vi "Write TAG (SubVI).vi"(11 "element":T1) -> (0 "error out":errorcluster)   [LabVIEW 2017]
uses:
  Vibration.ctl
  <vilib>/Skyline/Tag/Shared/typedefs/DataType.ctl
  <vilib>/Skyline/Tag/Wrapper/Wrapper AMQP_class/Open Tag AMQP.vi
  <vilib>/Skyline/Tag/Wrapper/Wrapper_class/Generate Tag Cluster (DBL) 2.vi
  <vilib>/Skyline/Tag/Wrapper/Wrapper_class/Generate Tag Cluster (Boolean) 2.vi
  <vilib>/Skyline/Tag/Wrapper/Wrapper_class/Close Tag (Multiple).vi
  <vilib>/Skyline/Tag/Shared/NI Skyline Tag.lvlib
  <vilib>/Skyline/Tag/Wrapper/Wrapper_class/NI Skyline Tag.lvclass
  <vilib>/Skyline/Tag/Wrapper/Wrapper AMQP_class/NI Skyline Tag AMQP.lvclass
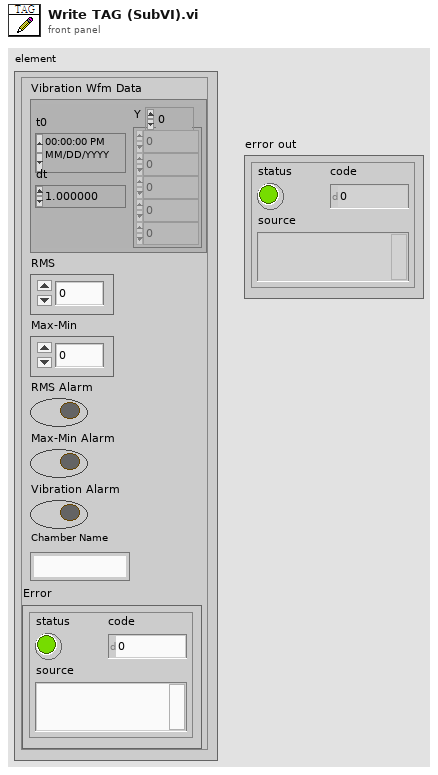
[diagram p1: front panel]
types:
  T1 = typedef "Vibration.ctl" = cluster{"Vibration Wfm Data":waveform(dbl), "RMS":dbl, "Max-Min":dbl, "RMS Alarm":bool, "Max-Min Alarm":bool, "Vibration Alarm":bool, "Chamber Name":string, "Error":errorcluster}
  T2 = typedef "NI Skyline Tag.lvlib/DataType.ctl" = enum32{"Double", "I32", "String", "Boolean", "U64", "Timestamp"}
  T3 = typedef "NI Skyline Tag.lvclass/Tag Value Cluster Wrapper.ctl" = cluster{"Configuration":refnum<class "NI Skyline Configuration.lvclass">, "Tag Cluster":T4}
  T4 = typedef "NI Skyline Tag.lvlib/Tag Value Cluster.ctl" = cluster{"Path":string, "Data Type":T2, "Value":string, "Time Stamp":timestamp}
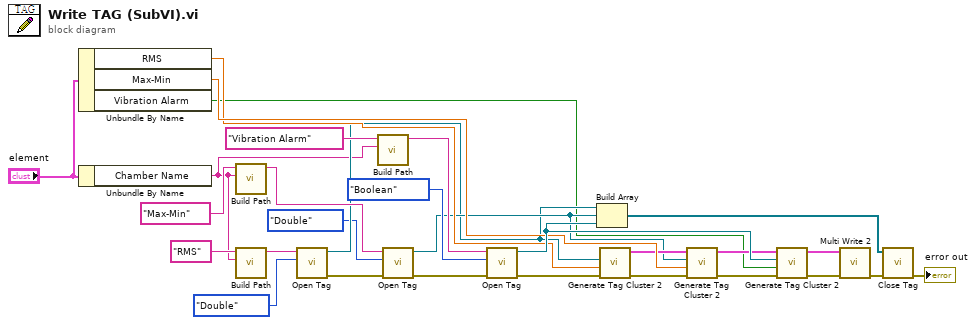
[diagram p0: block diagram]
diagram:
  n1 = Unbundle By Name("element") -> ("RMS"=w23:dbl, "Max-Min"=w24:dbl, "Vibration Alarm"=w6:bool)
  n2 = Unbundle By Name("element") -> ("Chamber Name"=w1:string)
  n3 = call <vilib>:"Build Path.vi"("namespace"=w1, "tag name"="Max-Min" ("tag path")) -> ("path"=w16:string)  [unwired: 9 in]
  n4 = call <vilib>:"Build Path.vi"("namespace"=w1, "tag name"="RMS" ("tag path")) -> ("path"=w5:string)  [unwired: 9 in]
  n5 = call-poly <vilib>:"Open Tag.vi"("data type"=DataType."Double" ("Data Type"), "path"=w5) -> ("error out"=w4:errorcluster, "tag out"=w11:refnum<class "NI Skyline Tag.lvclass">)  [unwired: 8 in]
  n6 = call <vilib>:"Build Path.vi"("namespace"=w1, "tag name"="Vibration Alarm" ("tag path")) -> ("path"=w18:string)  [unwired: 9 in]
  n7 = call-poly <vilib>:"Open Tag.vi"("error in (no error)"=w4, "data type"=DataType."Double" ("Data Type"), "path"=w16) -> ("error out"=w3:errorcluster, "tag out"=w13:refnum<class "NI Skyline Tag.lvclass">)  [unwired: 7 in]
  n8 = call-poly <vilib>:"Open Tag.vi"("error in (no error)"=w3, "data type"=DataType."Boolean" ("Data Type"), "path"=w18) -> ("error out"=w2:errorcluster, "tag out"=w29:refnum<class "NI Skyline Tag.lvclass">)  [unwired: 7 in]
  n9 = Build Array(w11, w13, w29) -> (w12:refnum<class "NI Skyline Tag.lvclass">[])
  n10 = call-poly <vilib>:"Generate Tag Cluster 2.vi"("error in (no error)"=w2, "value"=w23, "tag in"=w11) -> ("error out"=w21:errorcluster, "tag clusters out"=w22:T3[])  [unwired: 6 in, 1 out]
  n11 = call-poly <vilib>:"Generate Tag Cluster 2.vi"("error in (no error)"=w21, "value"=w24, "tag in"=w13, "tag clusters in"=w22) -> ("error out"=w26:errorcluster, "tag clusters out"=w25:T3[])  [unwired: 5 in, 1 out]
  n12 = call-poly <vilib>:"Generate Tag Cluster 2.vi"("error in (no error)"=w26, "value"=w6, "tag in"=w29, "tag clusters in"=w25) -> ("error out"=w28:errorcluster, "tag clusters out"=w27:T3[])  [unwired: 5 in, 1 out]
  n13 = call <vilib>:"Multi Write 2.vi"("error in (no error)"=w28, "tag clusters"=w27) -> ("error out"=w7:errorcluster)  [unwired: 9 in]
  n14 = call-poly <vilib>:"Close Tag.vi"("error in (no error)"=w7, "tags in"=w12) -> ("error out"=→"error out":errorcluster)  [unwired: 9 in]
